vi "RedlineOpenClimb.vi"   [LabVIEW 2020]
uses:
  <vilib>/Rock Robotics/WPI/ThirdParty/Phoenix-LabVIEW/Motor Controller/Controls/CTRE_Phoenix_MotorControl_NeutralMode.ctl
  <vilib>/Rock Robotics/WPI/Solenoid/WPI_SolenoidChannel.ctl
  <vilib>/Rock Robotics/WPI/Solenoid/WPI_SolenoidOpenDouble.vi
types:
  T1 = typedef "WPI_SolenoidChannel.ctl" = enum8{"Solenoid 0", "Solenoid 1", "Solenoid 2", "Solenoid 3", "Solenoid 4", "Solenoid 5", "Solenoid 6", "Solenoid 7", "Solenoid 8", "Solenoid 9", "Solenoid 10", "Solenoid 11", "Solenoid 12", "Solenoid 13", "Solenoid 14", "Solenoid 15", "Invalid"}
  T2 = typedef "CTRE_Phoenix_MotorControl_NeutralMode.ctl" = enum8{"EEPROMSetting", "Override to Coast", "Override to Brake"}
  T3 = typedef "WPI_MotorControlDeviceRef.ctl" = cluster{"DeviceStatus":errorcluster, "Type":T4, "PWM":cluster{"PWM Channel":T5, "DeadBand":T6}, "CAN":cluster{"Device Number":u8, "SetOutput VI Ref":variant, "GetOutput VI Ref":variant, "Enable VI Ref":variant, "Disable VI Ref":variant, "Data":variant}, "Invert":bool, "DIO PWM":cluster{"PWM \"Enable\" Channel":T5, "DIOChannel":T7, "PWM Rate":dbl}}
  T4 = typedef "WPI_MotorControlType.ctl" = enum16{"PWM", "CAN", "DIO PWM"}
  T5 = typedef "FPGA_DIOPWMChannel.ctl" = enum8{"PWM 0", "PWM 1", "PWM 2", "PWM 3", "PWM 4", "PWM 5", "PWM 6", "PWM 7", "PWM 8", "PWM 9", "PWM MXP 0", "PWM MXP 1", "PWM MXP 2", "PWM MXP 3", "PWM MXP 4", "PWM MXP 5", "PWM MXP 6", "PWM MXP 7", "PWM MXP 8", "PWM MXP 9", "Invalid"}
  T6 = typedef "WPI_PWMDeadband.ctl" = cluster{"Name":string, "maxPositivePwm":i32, "minPositivePwm":i32, "centerPwm":i32, "maxNegativePwm":i32, "minNegativePwm":i32, "angularRange":u16}
  T7 = typedef "FPGA_DIOChannel.ctl" = enum8{"DIO 0", "DIO 1", "DIO 2", "DIO 3", "DIO 4", "DIO 5", "DIO 6", "DIO 7", "DIO 8", "DIO 9", "DIO MXP 0", "DIO MXP 1", "DIO MXP 2", "DIO MXP 3", "DIO MXP 4", "DIO MXP 5", "DIO MXP 6", "DIO MXP 7", "DIO MXP 8", "DIO MXP 9", "DIO MXP 10", "DIO MXP 11", "DIO MXP 12", "DIO MXP 13", "DIO MXP 14", "DIO MXP 15", "SPI Port CS1", "SPI Port CS2", "SPI Port CS3", "SPI Port MISO", "SPI Port MOSI", "Invalid"}
  T8 = typedef "WPI_SolenoidDevRef.ctl" = cluster{"DevStatus":errorcluster, "Pneumatics Control Module":u8, "Forward Solenoid Channel":T1, "Reverse Solenoid Channel":T1}
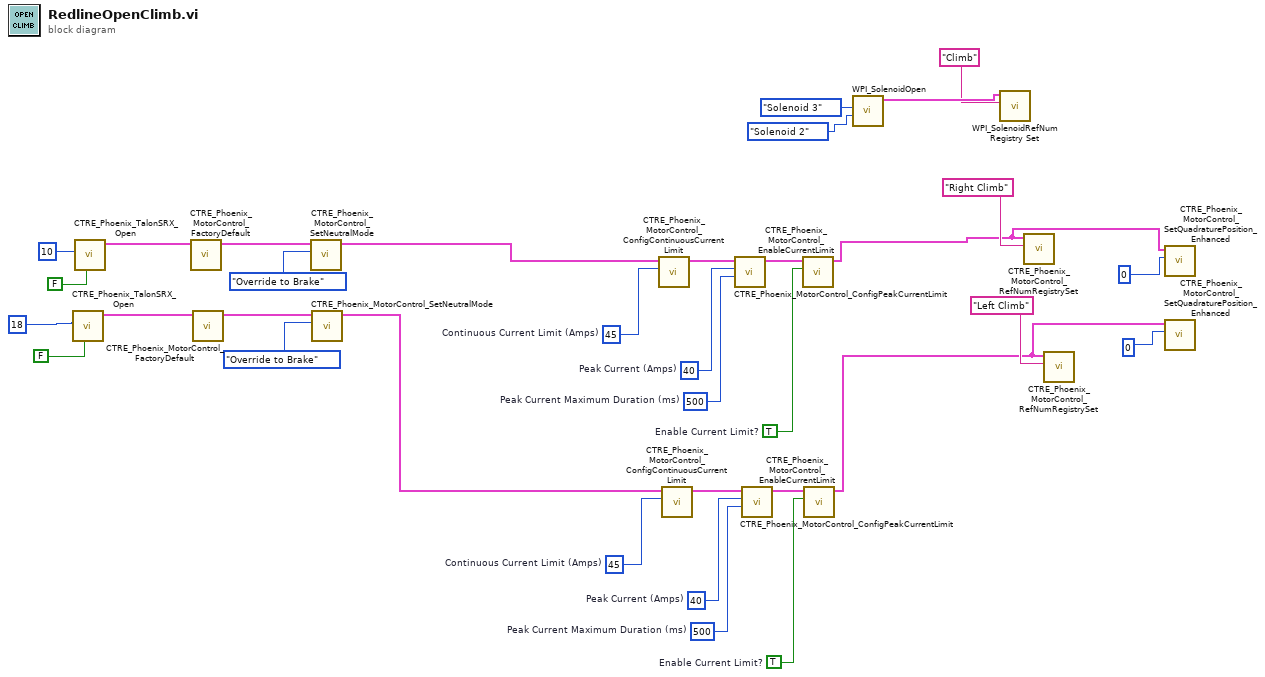
[diagram p0: block diagram]
diagram:
  w5 = TRUE  # Enable Current Limit?
  w8 = 500  # Peak Current Maximum Duration (ms)
  w9 = 40  # Peak Current (Amps)
  w10 = 45  # Continuous Current Limit (Amps)
  w11 = TRUE  # Enable Current Limit?
  w14 = 500  # Peak Current Maximum Duration (ms)
  w15 = 40  # Peak Current (Amps)
  w16 = 45  # Continuous Current Limit (Amps)
  n1 = call <vilib>:"CTRE_Phoenix_TalonSRX_Open.vi"("Invert"=FALSE, "Device Number"=u8 18) -> ("PhoenixMotorControlDevRef"=w25:T3)  [unwired: 8 in, 1 out]
  n2 = call <vilib>:"CTRE_Phoenix_TalonSRX_Open.vi"("Invert"=FALSE, "Device Number"=u8 10) -> ("PhoenixMotorControlDevRef"=w30:T3)  [unwired: 8 in, 1 out]
  n3 = call <vilib>:"CTRE_Phoenix_MotorControl_FactoryDefault.vi"("PhoenixMotorControlDevRef"=w30) -> ("PhoenixMotorControlDevRef"=w31:T3)  [unwired: 9 in, 1 out]
  n4 = call <vilib>:"CTRE_Phoenix_MotorControl_FactoryDefault.vi"("PhoenixMotorControlDevRef"=w25) -> ("PhoenixMotorControlDevRef"=w28:T3)  [unwired: 9 in, 1 out]
  n5 = call <vilib>:"CTRE_Phoenix_MotorControl_SetNeutralMode.vi"("Motor Control Neutral Mode"=CTRE_Phoenix_MotorControl_NeutralMode."Override to Brake", "PhoenixMotorControlDevRef"=w31) -> ("PhoenixMotorControlDevRef"=w4:T3)  [unwired: 8 in, 1 out]
  n6 = call <vilib>:"CTRE_Phoenix_MotorControl_SetNeutralMode.vi"("Motor Control Neutral Mode"=CTRE_Phoenix_MotorControl_NeutralMode."Override to Brake", "PhoenixMotorControlDevRef"=w28) -> ("PhoenixMotorControlDevRef"=w3:T3)  [unwired: 8 in, 1 out]
  n7 = call <vilib>:"CTRE_Phoenix_MotorControl_ConfigContinuousCurrentLimit.vi"("Continuous Current Limit (Amps)"=w10, "PhoenixMotorControlDevRef"=w4) -> ("PhoenixMotorControlDevRef"=w7:T3)  [unwired: 8 in, 1 out]
  n8 = call <vilib>:"CTRE_Phoenix_MotorControl_ConfigContinuousCurrentLimit.vi"("Continuous Current Limit (Amps)"=w16, "PhoenixMotorControlDevRef"=w3) -> ("PhoenixMotorControlDevRef"=w13:T3)  [unwired: 8 in, 1 out]
  n9 = call <vilib>:"CTRE_Phoenix_MotorControl_ConfigPeakCurrentLimit.vi"("Peak Current Maximum Duration (ms)"=w8, "Peak Current (Amps)"=w9, "PhoenixMotorControlDevRef"=w7) -> ("PhoenixMotorControlDevRef"=w6:T3)  [unwired: 7 in, 1 out]
  n10 = call <vilib>:"CTRE_Phoenix_MotorControl_ConfigPeakCurrentLimit.vi"("Peak Current Maximum Duration (ms)"=w14, "Peak Current (Amps)"=w15, "PhoenixMotorControlDevRef"=w13) -> ("PhoenixMotorControlDevRef"=w12:T3)  [unwired: 7 in, 1 out]
  n11 = call <vilib>:"CTRE_Phoenix_MotorControl_EnableCurrentLimit.vi"("Enable Current Limit?"=w5, "PhoenixMotorControlDevRef"=w6) -> ("PhoenixMotorControlDevRef"=w1:T3)  [unwired: 8 in, 1 out]
  n12 = call <vilib>:"CTRE_Phoenix_MotorControl_EnableCurrentLimit.vi"("Enable Current Limit?"=w11, "PhoenixMotorControlDevRef"=w12) -> ("PhoenixMotorControlDevRef"=w2:T3)  [unwired: 8 in, 1 out]
  n13 = call-poly <vilib>:"WPI_SolenoidOpen.vi"("Reverse Solenoid Channel"=WPI_SolenoidChannel."Solenoid 2" ("Solenoid Channel"), "Forward Solenoid Channel"=WPI_SolenoidChannel."Solenoid 3" ("Solenoid Channel")) -> ("SolenoidDevRef"=w21:T8)  [unwired: 8 in, 1 out]
  n14 = call <vilib>:"WPI_SolenoidRefNum Registry Set.vi"("refnum name"="Climb", "SolenoidDevRef"=w21) -> ()  [unwired: 8 in, 2 out]
  n15 = call <vilib>:"CTRE_Phoenix_MotorControl_RefNumRegistrySet.vi"("refnum name"="Right Climb", "PhoenixMotorControlDevRef"=w1) -> ()  [unwired: 8 in, 2 out]
  n16 = call <vilib>:"CTRE_Phoenix_MotorControl_RefNumRegistrySet.vi"("refnum name"="Left Climb", "PhoenixMotorControlDevRef"=w2) -> ()  [unwired: 8 in, 2 out]
  n17 = call <vilib>:"CTRE_Phoenix_MotorControl_SetQuadraturePosition_Enhanced.vi"("New Position"=0, "PhoenixMotorControlDevRef"=w1) -> ()  [unwired: 8 in, 2 out]
  n18 = call <vilib>:"CTRE_Phoenix_MotorControl_SetQuadraturePosition_Enhanced.vi"("New Position"=0, "PhoenixMotorControlDevRef"=w2) -> ()  [unwired: 8 in, 2 out]
